vi "Get App Data Folder Path.vi"(8 "error in (no error)":errorcluster) -> (0 "error out":errorcluster, 3 "Temp Folder Path":path)   [LabVIEW 2023, in "RFFixtureCharact.Public.lvlib"]
uses:
  RFFixtureCharact.Public.lvlib
  <vilib>/Utility/sysdir.llb/System Directory Type.ctl
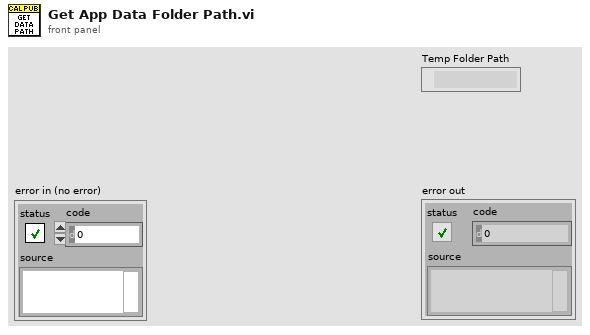
[diagram p1: front panel]
types:
  T1 = typedef "System Directory Type.ctl" = i32
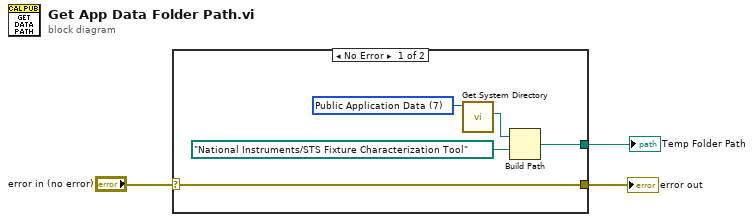
[diagram p0: block diagram]
diagram:
  n1 = case shown="No Error" "error in (no error)" {
    selector: "error in (no error)" -> [w4 w9]
    tunnel: [w5 _] -> w3
    tunnel: [w4 w9] -> w1
    frame No Error {
      w6 = T1 7 items=["User Home"=0, "User Desktop"=1, "User Documents"=2, "User Application Data"=3, "User Preferences"=4, "User Temporary"=5, "Public Documents"=6, "Public Application Data"=7, "Public Preferences"=8, "Public Cache"=13, "System Core Libraries"=9, "System Installed Libraries"=10, "Application Files"=11, "Boot Volume Root"=12] ("system directory type")
      n2 = call <vilib>:"Get System Directory.vi"("system directory type"=w6) -> ("system directory"=w7:path)  [unwired: 10 in]
      n3 = Build Path(base path=w7, name or relative path=path "National Instruments/STS Fixture Characterization Tool" ("Config File Relative Path")) -> (appended path=w5:path)
    }
    frame Error {
    }
  }
  "Temp Folder Path" <- w3
  "error out" <- w1
